vi "20151001 Data collect.vi"(5 "Epilson(Explore probability )":dbl min=0.0 max=1.0, 6 "Actions":i16[](array[numeric]), 8 "Error In":errorcluster, 9 "Pulse limit":T1, 10 "Sample set":T5, 11 "Neural Network in":T2={"Weigths"=[], "Last Layer Linear"=TRUE, "Add Bias Inputs"=TRUE, "# Inputs"=0, "# Output Neurons/Outputs"=0, "Inputs Scaling"={"X Scaling Vector"=[], "Y Scaling Vector"=[]}, "Outputs Scaling"={"X Scaling Vector"=[], "Y Scaling Vector"=[]}}) -> (0 "Error Out":errorcluster, 2 "Action":i16, 3 "Neural Network out":T2={"Weigths"=[], "Last Layer Linear"=TRUE, "Add Bias Inputs"=TRUE, "# Inputs"=0, "# Output Neurons/Outputs"=0, "Inputs Scaling"={"X Scaling Vector"=[], "Y Scaling Vector"=[]}, "Outputs Scaling"={"X Scaling Vector"=[], "Y Scaling Vector"=[]}})   [LabVIEW 2013]
uses:
  controls/Sample set.ctl
  SSNN(super simple neural network)_2.1/Neural Network/Types/Neural Network.ctl
  SSNN(super simple neural network)_2.1/Neural Network/Types/2D Array.ctl
  SSNN(super simple neural network)_2.1/Neural Network/Types/Scaling Info.ctl
  controls/Pulse limit.ctl
  <userlib>/_OpenG.lib/numeric/numeric.llb/Random Number Within Range - DBL__ogtk.vi
  <userlib>/_OpenG.lib/numeric/numeric.llb/Random Number Within Range - I32__ogtk.vi
  SSNN(super simple neural network)_2.1/Neural Network/Super Simple Neural Network.lvlib
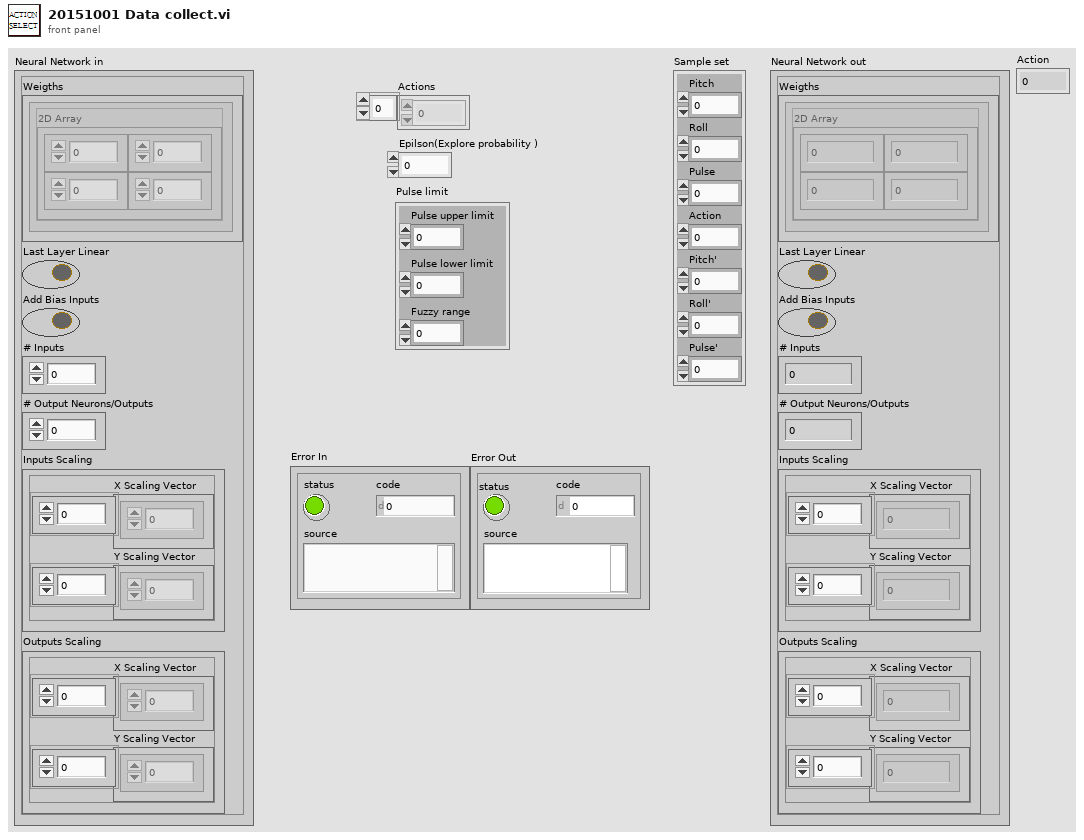
[diagram p1: front panel]
types:
  T1 = typedef "Pulse limit.ctl" = cluster{"Pulse upper limit":i16, "Pulse lower limit":i16, "Fuzzy range":dbl}
  T2 = typedef "Super Simple Neural Network.lvlib/Neural Network.ctl" = cluster{"Weigths":T3[], "Last Layer Linear":bool, "Add Bias Inputs":bool, "# Inputs":u32, "# Output Neurons/Outputs":u32, "Inputs Scaling":T4, "Outputs Scaling":T4}
  T3 = typedef "Super Simple Neural Network.lvlib/2D Array.ctl" = cluster{"2D Array":dbl[][]}
  T4 = typedef "Super Simple Neural Network.lvlib/Scaling Info.ctl" = cluster{"X Scaling Vector":dbl[], "Y Scaling Vector":dbl[]}
  T5 = typedef "Sample set.ctl" = cluster{"Pitch":dbl, "Roll":dbl, "Pulse":dbl, "Action":dbl, "Pitch'":dbl, "Roll'":dbl, "Pulse'":dbl}
  T6 = cluster{"LLR Act":i16[], "ULR Act":i16[], "In range Act":i16[]}
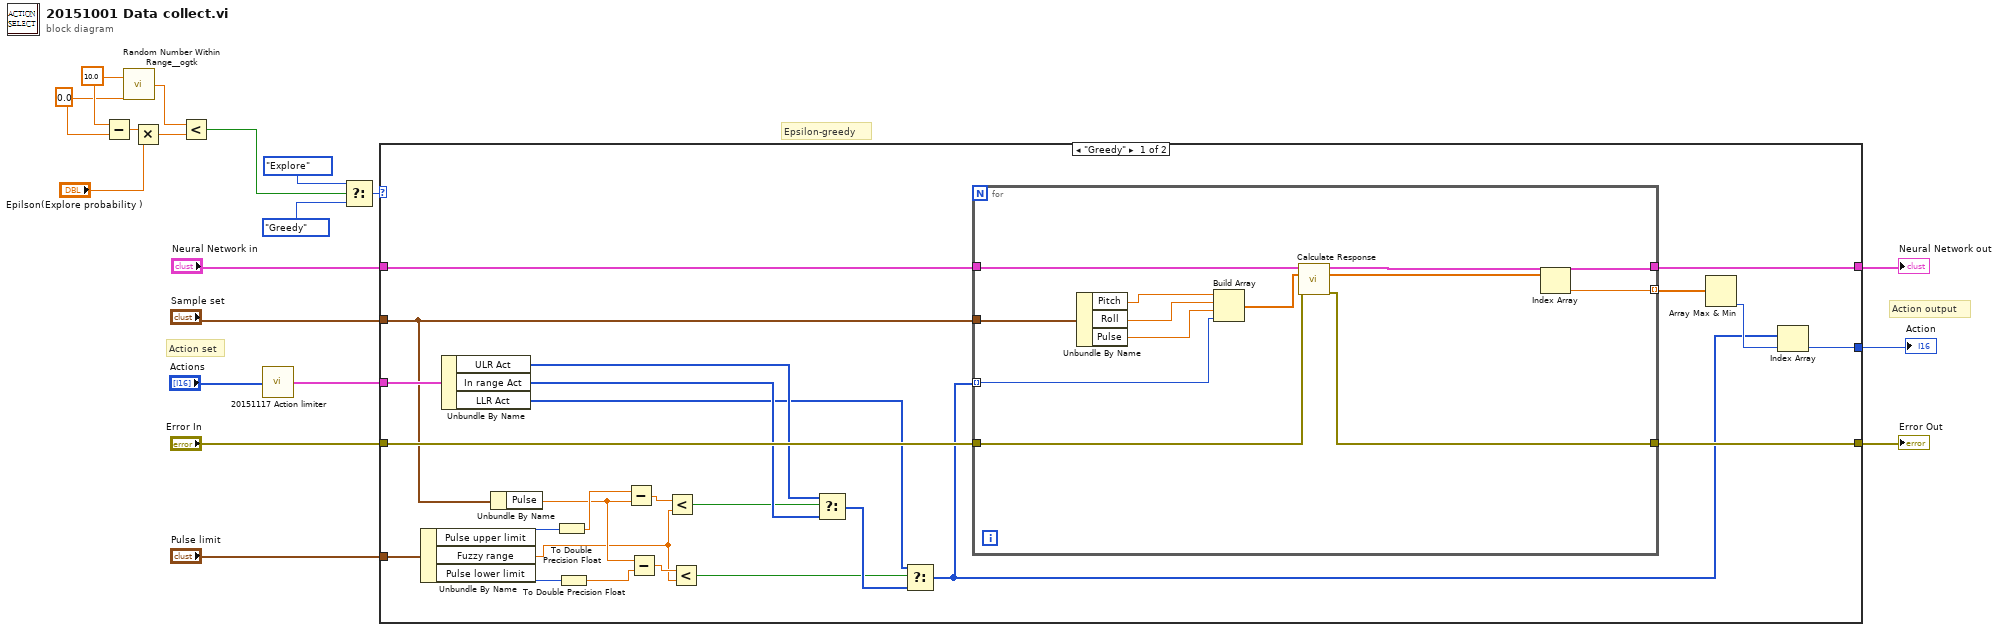
[diagram p0: block diagram]
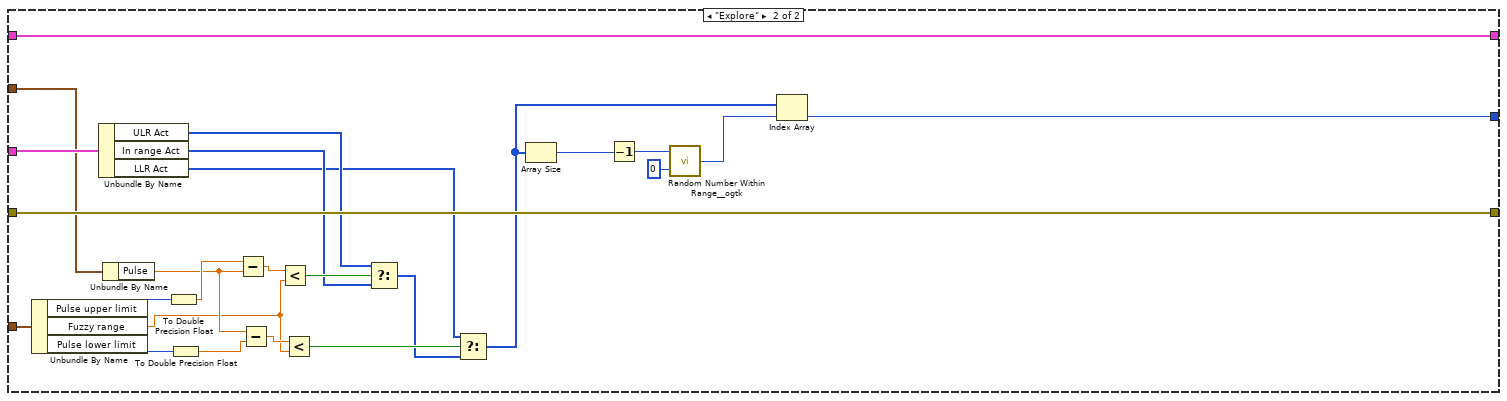
[diagram p2: hidden frame]
diagram:
  w15 = 0.0 ("Low")
  w16 = 10.0 ("High")
  # "Action set"
  # "Epsilon-greedy"
  # "Action output"
  n1 = Subtract(x=w16, y=w15) -> (x-y=w17:dbl)
  n2 = call-poly <userlib>:"Random Number Within Range__ogtk.vi"("High"=w16, "Low"=w15) -> ("Random Number"=w19:dbl)  [unwired: 3 in]
  n3 = Multiply(x=w17, y="Epilson(Explore probability )") -> (x*y=w18:dbl)
  n4 = Less?(x=w19, y=w18) -> (x < y?=w12:bool)
  n5 = call "20151117 Action limiter.vi"("Actions"="Actions") -> ("Action limiter"=w1:T6)  [unwired: 4 in]
  n6 = Select(t=enum16{"Greedy", "Explore"}."Explore", s=w12, f=enum16{"Greedy", "Explore"}."Greedy") -> (s? t:f=w13:enum16{"Greedy", "Explore"})
  n7 = case shown="\"Greedy\"" w13 {
    tunnel: "Sample set" -> [w23 w66]
    tunnel: [w44 w64] -> w5
    tunnel: "Neural Network in" -> [w43 w76]
    tunnel: "Error In" -> [w42 w77]
    tunnel: [w41 w77] -> w8
    tunnel: [w40 w76] -> w7
    tunnel: "Pulse limit" -> [w22 w68]
    tunnel: w1 -> [w36 w67]
    frame "Greedy" {
      n8 = Unbundle By Name(w22) -> ("Pulse upper limit"=w31:i16, "Fuzzy range"=w24:dbl, "Pulse lower limit"=w25:i16)
      n9 = Unbundle By Name(w36) -> ("ULR Act"=w35:i16[], "In range Act"=w34:i16[], "LLR Act"=w33:i16[])
      n10 = Unbundle By Name(w23) -> ("Pulse"=w27:dbl)
      n11 = To Double Precision Float(number=w31) -> (double precision float=w29:dbl)
      n12 = To Double Precision Float(number=w25) -> (double precision float=w26:dbl)
      n13 = Subtract(x=w29, y=w27) -> (x-y=w30:dbl)
      n14 = Subtract(x=w27, y=w26) -> (x-y=w28:dbl)
      n15 = Less?(x=w30, y=w24) -> (x < y?=w21:bool)
      n16 = Less?(x=w28, y=w24) -> (x < y?=w20:bool)
      n17 = Select(t=w35, s=w21, f=w34) -> (s? t:f=w39:i16[])
      n18 = Select(t=w33, s=w20, f=w39) -> (s? t:f=w32:i16[])
      n19 = for {
        tunnel: w23 -> [w56]
        tunnel: w32 -> [w48] mode=indexing
        tunnel: [w52] -> w37 mode=indexing
        tunnel: w43 -> [w51]
        tunnel: w42 -> [w50]
        tunnel: [w49] -> w41
        tunnel: [w46] -> w40
        n20 = Unbundle By Name(w56) -> ("Pitch"=w54:dbl, "Roll"=w53:dbl, "Pulse"=w47:dbl)
        n21 = Build Array(w54, w53, w47, w48) -> (w55:dbl[])
        n22 = call "Calculate Response.vi"("Neural Network In"=w51, "Inputs"=w55, "Error In"=w50) -> ("Neural Network Out"=w46:T2, "Outputs"=w45:dbl[], "Error Out"=w49:errorcluster)  [unwired: 10 in]
        n23 = Index Array(array=w45) -> (element=w52:dbl)  [unwired: 1 in]
      }
      n24 = Array Max & Min(array=w37) -> (min index (indices)=w38:i32)  [unwired: 3 out]
      n25 = Index Array(array=w32, index=w38) -> (element=w44:i16)
    }
    frame "Explore" {
      n26 = Unbundle By Name(w68) -> ("Pulse upper limit"=w69:i16, "Fuzzy range"=w57:dbl, "Pulse lower limit"=w58:i16)
      n27 = Unbundle By Name(w67) -> ("ULR Act"=w72:i16[], "In range Act"=w71:i16[], "LLR Act"=w70:i16[])
      n28 = Unbundle By Name(w66) -> ("Pulse"=w60:dbl)
      n29 = To Double Precision Float(number=w69) -> (double precision float=w62:dbl)
      n30 = To Double Precision Float(number=w58) -> (double precision float=w59:dbl)
      n31 = Subtract(x=w62, y=w60) -> (x-y=w63:dbl)
      n32 = Subtract(x=w60, y=w59) -> (x-y=w61:dbl)
      n33 = Less?(x=w63, y=w57) -> (x < y?=w75:bool)
      n34 = Less?(x=w61, y=w57) -> (x < y?=w74:bool)
      n35 = Select(t=w72, s=w75, f=w71) -> (s? t:f=w73:i16[])
      n36 = Select(t=w70, s=w74, f=w73) -> (s? t:f=w65:i16[])
      n37 = Array Size(array=w65) -> (size(s)=w80:i32)
      n38 = Decrement(x=w80) -> (x-1=w79:i32)
      n39 = call-poly <userlib>:"Random Number Within Range__ogtk.vi"("High"=w79, "Low"=0) -> ("Random Number"=w78:i32)  [unwired: 3 in]
      n40 = Index Array(array=w65, index=w78) -> (element=w64:i16)
    }
  }
  "Error Out" <- w8
  "Neural Network out" <- w7
  "Action" <- w5
